vi "SaveFileToMIDAS.vi"(9 "Filename":string, 10 "Project Name":string, 11 "File":path) -> (1 "MD5 message-digest":string, 2 "MD5 Error out":errorcluster, 3 "Log This Error Out":errorcluster)   [LabVIEW 2018, in "feGEM DataPacker.lvlib"]
uses:
  feGEM DataPacker.lvlib
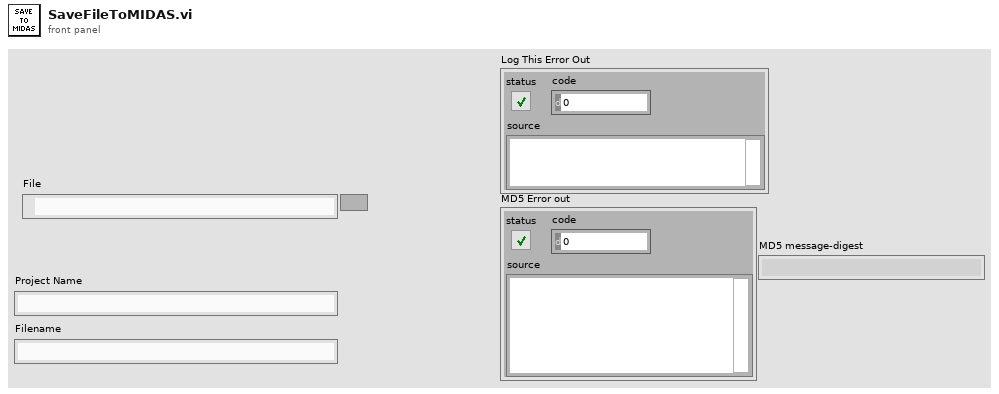
[diagram p1: front panel]
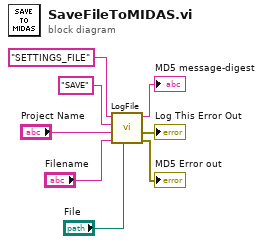
[diagram p0: block diagram]
diagram:
  n1 = call "LogFile.vi"("File"="File", "Filename (optional)"="Filename", "Project Name (Unlimited length... Key word for analyzer, or folder for MIDAS settings file database)"="Project Name", "Variable name (SAVE and LOAD are magic keywords for the MIDAS settings file database)"="SAVE", "Category (SETTINGS_FILE is a magic keyword for the MIDAS settings file database)"="SETTINGS_FILE") -> ("MD5 Error out"=→"MD5 Error out":errorcluster, "Log This Error Out"=→"Log This Error Out":errorcluster, "MD5 message-digest"=→"MD5 message-digest":string)  [unwired: 4 in]
